vi "LV to ITX  Retrieve_SE mode  calculate R.vi"(0 "File or Folder Path":path=path "\\\\WINDYSEA\\Data/SA02835E.20160621/5_IV - sweep Bx, By, Vsg", 5 "offset":i32, 7 "length":i32=1, 9 "index":T2={"A"=3, "B"=7, "C"=5, "D"=7, "E"=3, "N1"=22, "N2"=2, "N3"=3, "N4"=4, "A 1"=8, "A 2"=10, "C 1"=5, "C 2"=1, "E 2"=4}, 11 "stop":bool=TRUE, 12 "file contains 2D data?":bool) -> (1 "Spherical coordinates":dbl[][](array[numeric]), 2 "long":cluster{i32[], dbl[]}(graph), 3 "G vs T":cluster{dbl[], dbl[]}(graph), 4 "A vs B":cluster{dbl[], dbl[]}[](graph), 6 "C vs D":cluster{dbl[], dbl[]}[](graph), 8 "E( = A)":dbl[][](graph), 10 "N":cluster{"N1":dbl, "N2":dbl, "N3":dbl, "N4":dbl}={"N1"=0.275, "N2"=1.998590895326537, "N3"=1.188236459055352e-05, "N4"=3.553800592300099e-05} {"N4" format="%#_6p"; "N3" format="%#_6p"; "N2" format="%#_6p"; "N1" format="%#_6p"}, 13 "Index, Wavenames":string[][](table)=[["0", "'time.SA02835E.20160621.000000'\n"], ["1", "'temp.SA02835E.20160621.000000'\n"], ["2", "'Bx.SA02835E.20160621.000000'\n"], ["3", "'By.SA02835E.20160621.000000'\n"], ["4", "'Bz.SA02835E.20160621.000000'\n"], ["5", "'Vsource.SA02835E.20160621.000000'\n"], ["6", "'Lockin0.SA02835E.20160621.000000'\n"], ["7", "'Lockin1.SA02835E.20160621.000000'\n"], ["8", "'Lockin2.SA02835E.20160621.000000'\n"], ["9", "'Lockin3.SA02835E.20160621.000000'\n"], ["10", "'Lockin4.SA02835E.20160621.000000'\n"], ["11", "'Lockin5.SA02835E.20160621.000000'\n"], ["12", "'Lockin6.SA02835E.20160621.000000'\n"], ["13", "'Lockin7.SA02835E.20160621.000000'\n"], ["14", "'B_rate.SA02835E.20160621.000000'\n"], ["15", "'DC0.SA02835E.20160621.000000'\n"], ["16", "'DC1.SA02835E.20160621.000000'\n"], ["17", "'DC2.SA02835E.20160621.000000'\n"], ["18", "'DC3.SA02835E.20160621.000000'\n"], ["19", "'DC4.SA02835E.20160621.000000'\n"], ["20", "'DC5.SA02835E.20160621.000000'\n"], ["21", "'DC6.SA02835E.20160621.000000'\n"], ["22", "'DC7.SA02835E.20160621.000000'\n"], ["23", "'V4T.SA02835E.20160621.000000'\n"], ["24", "'I.SA02835E.20160621.000000'\n"], ["", ""]], 14 "Comments":string="IGOR\nX// Date: 6/25/2016 8:10 PM\nX// sweep in plane: from theta=0 deg to 360 deg in 10 deg steps (phi=90, xy plane) @ 0.005 T/min\nX// sweep Vsg: -30mV to 275mV, 1mV steps\nX// \nX// taking lockin data between Bfield setpoints\nX// \nX// IV:\nX// low cutoff f: 0.01\nX// decimate: 10\nX// \nX// Vbg=0.57V\nX// \nX// lockin:\nX// 0: 27\nX// 1: 1 current, 3mV AC, 675uV DC, 0.4Hz\nX// 2: 2, \nX// 3: 6,\nX// 4: 7 \nX// 5: 8 current\nX// 6; 28 \nX// appliedVsg= -0.030000\n\n\n\n\n\n\n\n\n\n\n\n\n\n\n\n\n\n\n\n\n\n\n\n\n\n\n\n\n\n\n\n\n\n\n\n\n\n\n\n\n\n\n\n\n\n\n\n\n\n\n\n\nX \nX Display/R 'time.SA02835E.20160621.000000'\nX AppendToGraph 'temp.SA02835E.20160621.000000'\nX AppendToGraph 'Bx.SA02835E.20160621.000000'\nX AppendToGraph 'By.SA02835E.20160621.000000'\nX AppendToGraph 'Bz.SA02835E.20160621.000000'\nX AppendToGraph 'Vsource.SA02835E.20160621.000000'\nX AppendToGraph 'Lockin0.SA02835E.20160621.000000'\nX AppendToGraph 'Lockin1.SA02835E.20160621.000000'\nX AppendToGraph 'Lockin2.SA02835E.20160621.000000'\nX AppendToGraph 'Lockin3.SA02835E.20160621.000000'\nX AppendToGraph 'Lockin4.SA02835E.20160621.000000'\nX AppendToGraph 'Lockin5.SA02835E.20160621.000000'\nX AppendToGraph 'Lockin6.SA02835E.20160621.000000'\nX AppendToGraph 'Lockin7.SA02835E.20160621.000000'\nX AppendToGraph 'B_rate.SA02835E.20160621.000000'\nX AppendToGraph 'DC0.SA02835E.20160621.000000'\nX AppendToGraph 'DC1.SA02835E.20160621.000000'\nX AppendToGraph 'DC2.SA02835E.20160621.000000'\nX AppendToGraph 'DC3.SA02835E.20160621.000000'\nX AppendToGraph 'DC4.SA02835E.20160621.000000'\nX AppendToGraph 'DC5.SA02835E.20160621.000000'\nX AppendToGraph 'DC6.SA02835E.20160621.000000'\nX AppendToGraph 'DC7.SA02835E.20160621.000000'\nX AppendToGraph 'V4T.SA02835E.20160621.000000'\nX AppendToGraph 'I.SA02835E.20160621.000000'\nX Label bottom \"x label\"\nX Label left \"y label\"\nX ModifyGraph rgb('time.SA02835E.20160621.000000')=(65280,0,0)\nX ModifyGraph rgb('temp.SA02835E.20160621.000000')=(65280,13824,0)\nX ModifyGraph rgb('Bx.SA02835E.20160621.000000')=(65280,27648,0)\nX ModifyGraph rgb('By.SA02835E.20160621.000000')=(65280,43008,0)\nX ModifyGraph rgb('Bz.SA02835E.20160621.000000')=(65280,56832,0)\nX ModifyGraph rgb('Vsource.SA02835E.20160621.000000')=(60416,65280,0)\nX ModifyGraph rgb('Lockin0.SA02835E.20160621.000000')=(46592,65280,0)\nX ModifyGraph rgb('Lockin1.SA02835E.20160621.000000')=(32768,65280,0)\nX ModifyGraph rgb('Lockin2.SA02835E.20160621.000000')=(17408,65280,0)\nX ModifyGraph rgb('Lockin3.SA02835E.20160621.000000')=(3584,65280,0)\nX ModifyGraph rgb('Lockin4.SA02835E.20160621.000000')=(0,65280,10240)\nX ModifyGraph rgb('Lockin5.SA02835E.20160621.000000')=(0,65280,24064)\nX ModifyGraph rgb('Lockin6.SA02835E.20160621.000000')=(0,65280,37888)\nX ModifyGraph rgb('Lockin7.SA02835E.20160621.000000')=(0,65280,53248)\nX ModifyGraph rgb('B_rate.SA02835E.20160621.000000')=(0,64000,65280)\nX ModifyGraph rgb('DC0.SA02835E.20160621.000000')=(0,50176,65280)\nX ModifyGraph rgb('DC1.SA02835E.20160621.000000')=(0,36352,65280)\nX ModifyGraph rgb('DC2.SA02835E.20160621.000000')=(0,22528,65280)\nX ModifyGraph rgb('DC3.SA02835E.20160621.000000')=(0,7168,65280)\nX ModifyGraph rgb('DC4.SA02835E.20160621.000000')=(6656,0,65280)\nX ModifyGraph rgb('DC5.SA02835E.20160621.000000')=(20480,0,65280)\nX ModifyGraph rgb('DC6.SA02835E.20160621.000000')=(34304,0,65280)\nX ModifyGraph rgb('DC7.SA02835E.20160621.000000')=(48128,0,65280)\nX ModifyGraph rgb('V4T.SA02835E.20160621.000000')=(63488,0,65280)\nX ModifyGraph rgb('I.SA02835E.20160621.000000')=(65280,0,53760)\nX Legend/C/N=text0/J \"\\\\s('time.SA02835E.20160621.000000') time\\r\\\\s('temp.SA02835E.20160621.000000') temp\\r\\\\s('Bx.SA02835E.20160621.000000') Bx\\r\\\\s('By.SA02835E.20160621.000000') By\\r\\\\s('Bz.SA02835E.20160621.000000') Bz\\r\\\\s('Vsource.SA02835E.20160621.000000') Vsource\\r\\\\s('Lockin0.SA02835E.20160621.000000') Lockin0\\r\\\\s('Lockin1.SA02835E.20160621.000000') Lockin1\\r\\\\s('Lockin2.SA02835E.20160621.000000') Lockin2\\r\\\\s('Lockin3.SA02835E.20160621.000000') Lockin3\\r\\\\s('Lockin4.SA02835E.20160621.000000') Lockin4\\r\\\\s('Lockin5.SA02835E.20160621.000000') Lockin5\\r\\\\s('Lockin6.SA02835E.20160621.000000') Lockin6\\r\\\\s('Lockin7.SA02835E.20160621.000000') Lockin7\\r\\\\s('B_rate.SA02835E.20160621.000000') B_rate\\r\\\\s('DC0.SA02835E.20160621.000000') DC0\\r\\\\s('DC1.SA02835E.20160621.000000') DC1\\r\\\\s('DC2.SA02835E.20160621.000000') DC2\\r\\\\s('DC3.SA02835E.20160621.000000') DC3\\r\\\\s('DC4.SA02835E.20160621.000000') DC4\\r\\\\s('DC5.SA02835E.20160621.000000') DC5\\r\\\\s('DC6.SA02835E.20160621.000000') DC6\\r\\\\s('DC7.SA02835E.20160621.000000') DC7\\r\\\\s('V4T.SA02835E.20160621.000000') V4T\\r\\\\s('I.SA02835E.20160621.000000') I\"\nX ModifyGraph mirror(bottom)=1\nX ModifyGraph width=216\nX ModifyGraph height={Aspect,0.6}\nX ModifyGraph Log(bottom)=0\nX ModifyGraph Log(left)=0\nX \n", 15 "E index vs Field":cluster{i32[], dbl[]}(graph))   [LabVIEW 2016]
uses:
  <vilib>/Utility/miscctls.llb/LVOffsetAndMultiplierTypeDef.ctl
  <vilib>/Analysis/3filter.llb/Savitzky-Golay Filter (DBL).vi
  <vilib>/Analysis/2dsp.llb/Decimate (single shot, DBL).vi
  <vilib>/Analysis/NI_AALPro.lvlib
  <vilib>/Analysis/NI_AALBase.lvlib
panel:
  out "A or C vs N3":cluster{dbl[], dbl[]}[](graph)
  in  "A":bool
  in  "VRM mode":bool
  in  "Ring":u16(ring) items=["default", "DIFF"]
  in  "decimating factor":i32=1
  in  "decimate files":i32=1
  in  "side points":i32=6
  in  "fit points":dbl=10.0
  in  "dy/dx vs x":bool=TRUE
  in  "Portion of data":cluster{dbl, dbl}(slide)={0.75, 0.25} scale=0.0..1.0
  in  "length 2":i32=498
  in  "index 2":i32=72
  out "Ns":T1(array[cluster])
  in  "SE?":bool=TRUE
  in  "D  is time?":bool
  in  "B is time?":bool
  out "time":string[][](table)=[["6/25/2016", "8:10 PM"]]
  in  "Use Folder Index File?":bool
  in  "Generate Folder Index File?":bool
  in  "Ez name":string="Conductance (S)"
  in  "Ey name":string="BY (T)"
  in  "Ex name":string="Vsg (mV)"
  in  "C y name":string="voltage"
  in  "D x name":string="Vsg"
  in  "A y name":string="current"
  in  "B x name":string="Vsg"
  in  "recolor traces?":bool
  in  "Ex":T3={"Offset"=0.0, "Multiplier"=1.0}
  in  "Ey":T3={"Offset"=0.0, "Multiplier"=1.0}
  out "Path":path=path "\\\\WINDYSEA\\Data/SA02835E.20160621/5_IV - sweep Bx, By, Vsg/SA02835E.20160621.000000.itx"
  out "counter":i32
  in  "pattern":string="*.itx"
  # "A1-A2\nC1-C2\nE-E2"
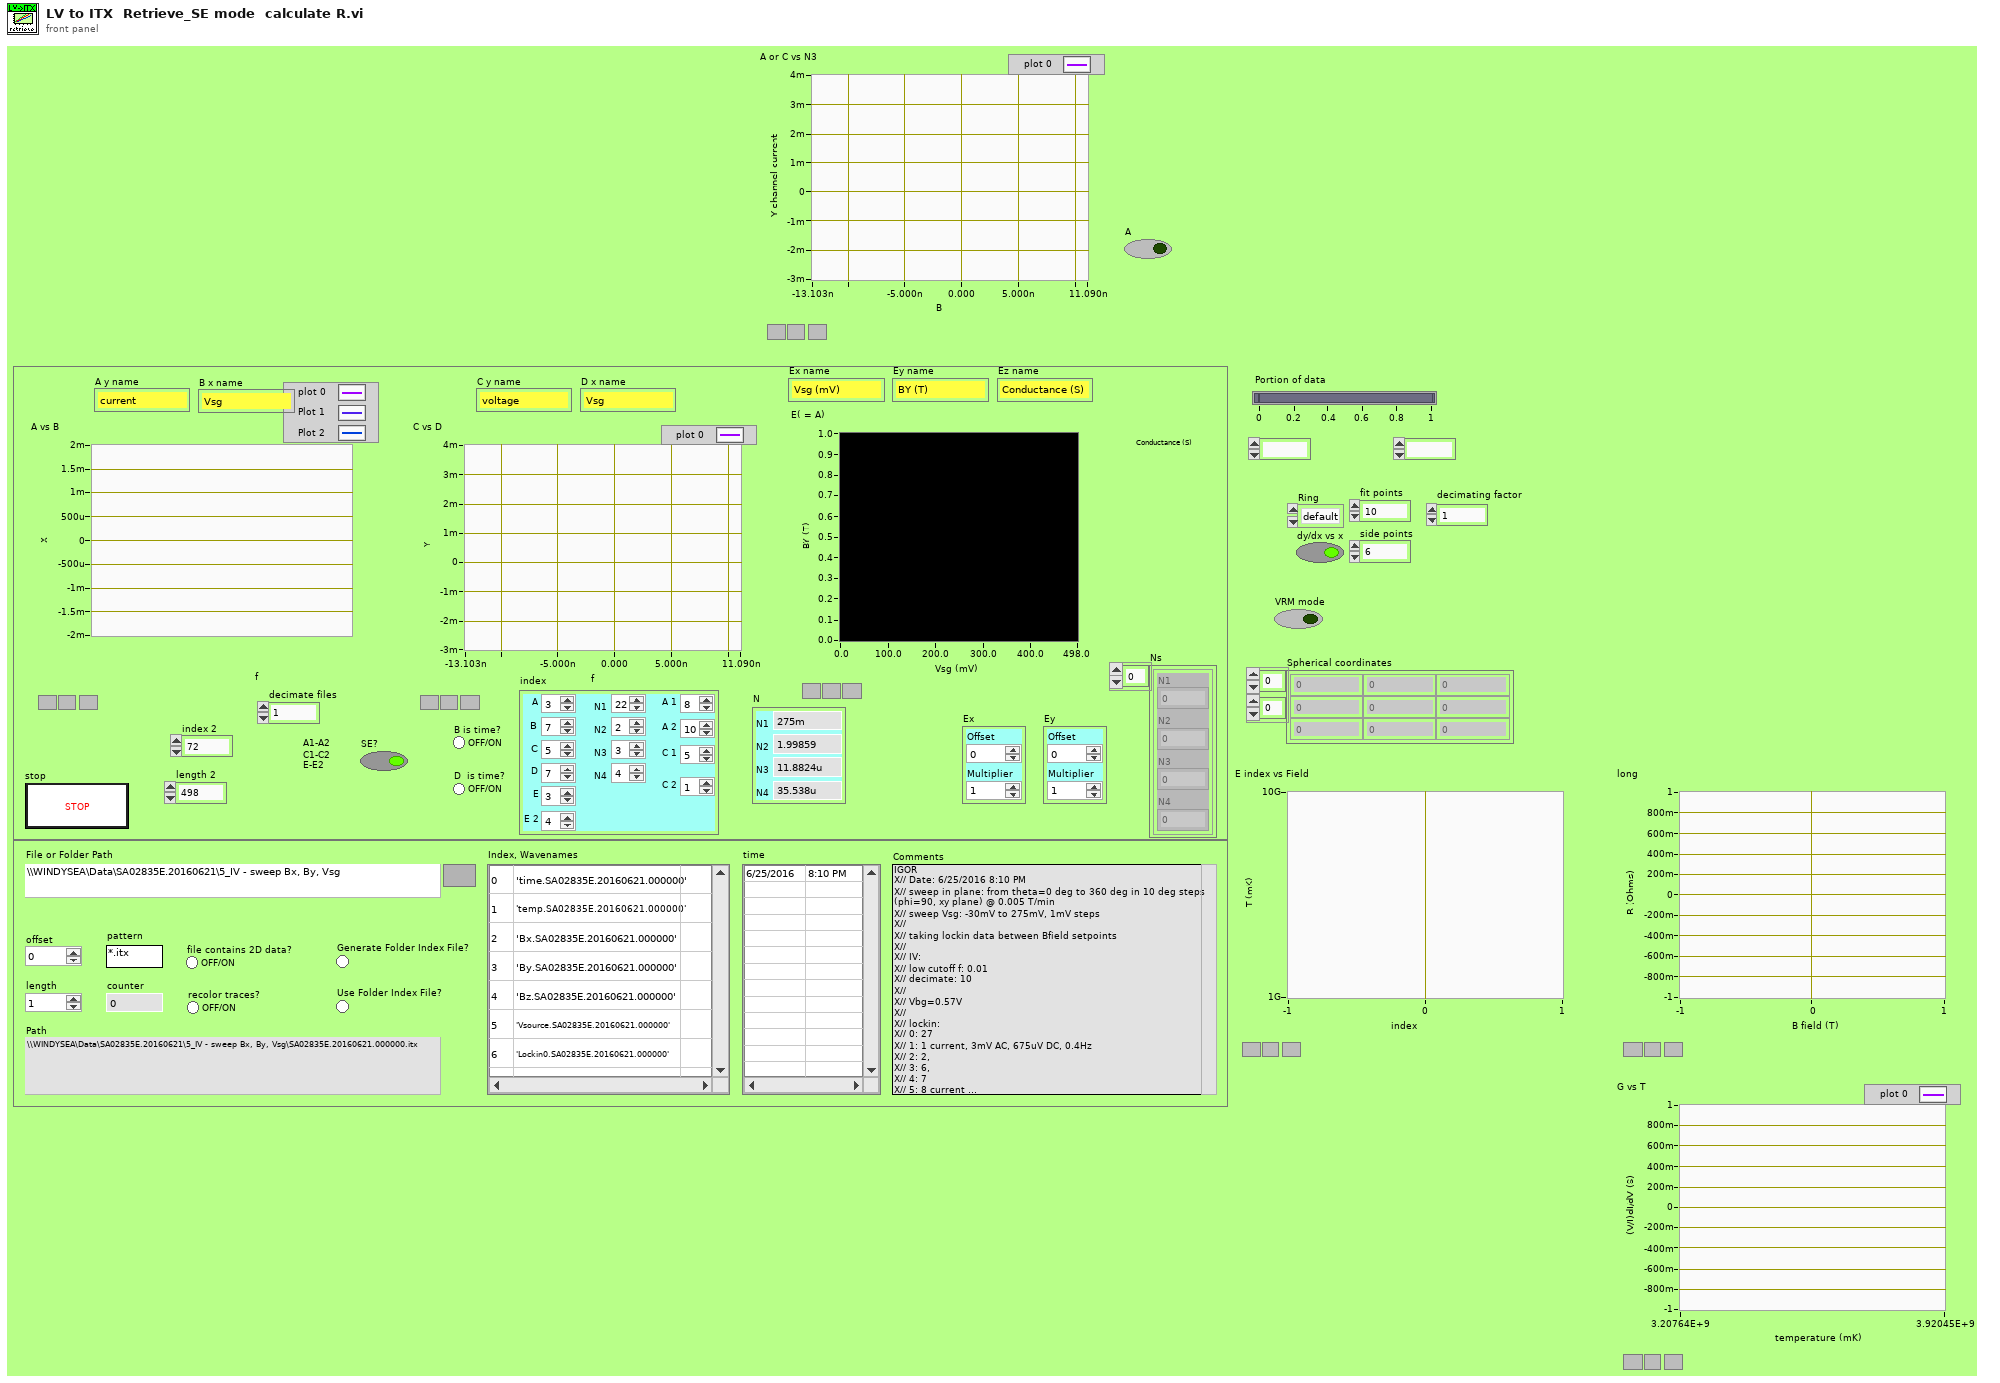
[diagram p1: front panel]
types:
  T1 = cluster{"N1":dbl, "N2":dbl, "N3":dbl, "N4":dbl}[]
  T2 = cluster{"A":i32, "B":i32, "C":i32, "D":i32, "E":i32, "N1":i32, "N2":i32, "N3":i32, "N4":i32, "A 1":i32, "A 2":i32, "C 1":i32, "C 2":i32, "E 2":i32}
  T3 = typedef "LVOffsetAndMultiplierTypeDef.ctl" = cluster{"Offset":dbl, "Multiplier":dbl}
  T4 = cluster{"Decimated Array":dbl[], "Decimated Array":dbl[]}
  T5 = cluster{"Decimated Array":dbl[], "Filtered X":dbl[]}
  T6 = cluster{"Decimated Array":dbl[], "Filtered X":dbl[]}[]
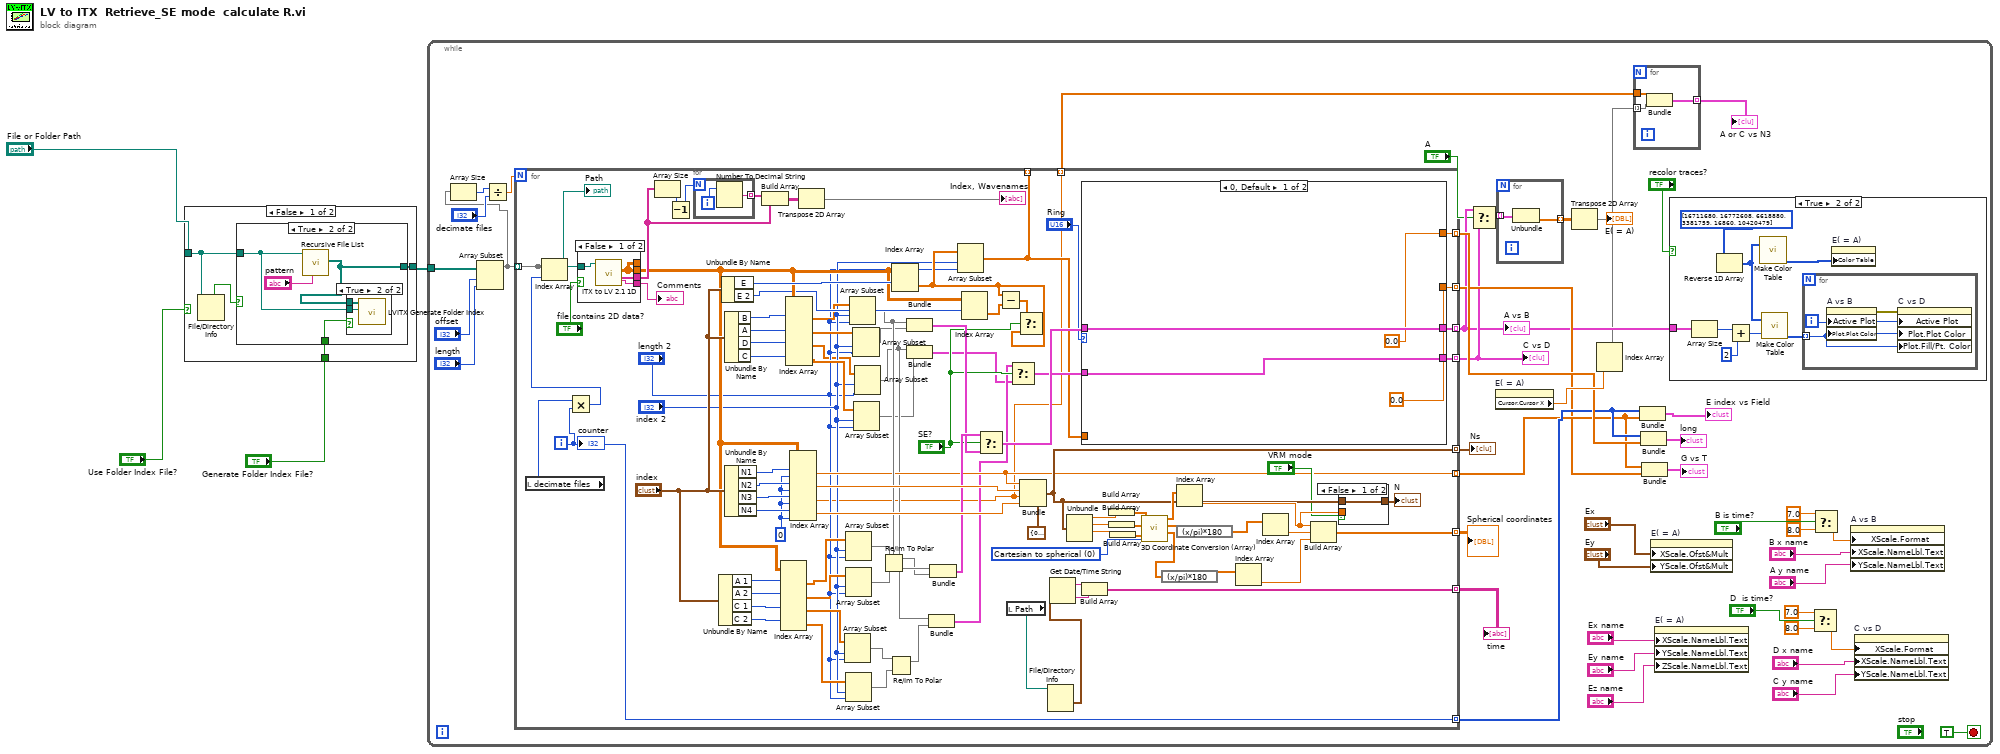
[diagram p0: block diagram]
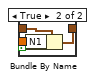
[diagram p3: hidden frame]
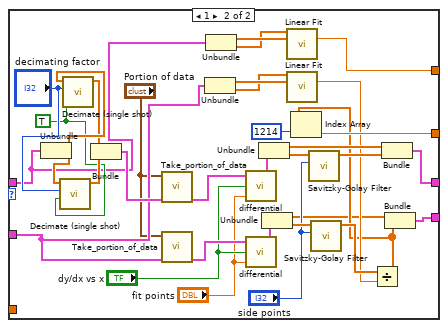
[diagram p4: hidden frame]
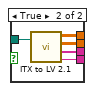
[diagram p5: hidden frame]
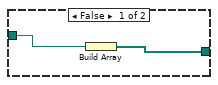
[diagram p6: hidden frame]
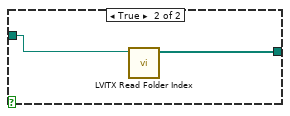
[diagram p8: hidden frame]
diagram:
  n1 = case shown="False" "Use Folder Index File?" {
    tunnel: [w6 w17] -> w2
    tunnel: "File or Folder Path" -> [w8 w18]
    tunnel: "Generate Folder Index File?" -> [w5 _]
    frame False {
      n2 = File/Directory Info(path=w8) -> (directory=w7:bool)  [unwired: 1 in, 6 out]
      n3 = case shown="True" w7 {
        tunnel: [w10 w13] -> w6
        tunnel: w8 -> [w9 w12]
        tunnel: w5 -> [_ w11]
        frame False {
          n4 = Build Array(w9) -> (w10:path[])
        }
        frame True {
          n5 = call <vilib>:"Recursive File List.vi"("pattern"="pattern", "Folder Path"=w12) -> ("All Files in Dir"=w13:path[])  [unwired: 5 in, 4 out]
          n6 = case shown="True" w11 {
            tunnel: w13 -> [_ w16]
            tunnel: w12 -> [_ w15]
            frame False {
            }
            frame True {
              n7 = call <userlib>:"LVITX Generate Folder Index.vi"("File or Folder Path"=w15, "All Files in Dir"=w16) -> ()  [unwired: 10 in]
            }
          }
        }
      }
    }
    frame True {
      n8 = call <userlib>:"LVITX Read Folder Index.vi"("File or Folder Path"=w18) -> ("Array"=w17:path[])  [unwired: 10 in]
    }
  }
  n9 = while {
    tunnel: w2 -> [w40]
    stop <- TRUE stop-if-true
    n10 = Array Subset(array=w40, index="offset", length="length") -> (w36:path[])
    n11 = Array Size(array=w36) -> (size(s)=w39:i32)
    n12 = Divide(x=w39, y="decimate files") -> (x/y=w37:dbl)
    n13 = for {
      N: w37 -> [_]
      tunnel: w36 -> [w173]
      tunnel: [w173] -> _ mode=indexing
      tunnel: [w111] -> w23 mode=indexing
      tunnel: [w110] -> w24 mode=indexing
      tunnel: [w149] -> w54 mode=indexing
      tunnel: [w100] -> w43 mode=indexing
      tunnel: [w109] -> w41 mode=indexing
      tunnel: [w103] -> w33 mode=indexing
      tunnel: [w102] -> w26 mode=indexing
      tunnel: [w97] -> w29 mode=indexing
      tunnel: [w96] -> w28 mode=indexing
      tunnel: [w81] -> _ mode=indexing
      tunnel: [w80] -> w20 mode=indexing
      i -> [w97]
      w126 = u16 0 items=["Cartesian to spherical", "spherical to Cartesian", "Cartesian to cylindrical", "cylindrical to Cartesian", "spherical to cylindrical", "cylindrical to spherical"] ("conversion type")
      w147 = 0 ("disabled index (col)")
      n14 = local read "decimate files"() -> (w106:i32)
      n15 = Multiply(x=w106, y=w97) -> (x*y=w107:i32)
      n16 = Index Array(array=w173, index=w107) -> (element=w108:path)
      "Path" <- w108
      n17 = case shown="False" "file contains 2D data?" {
        tunnel: [w222 w225] -> w174
        tunnel: [w220 w226] -> w139
        tunnel: w108 -> [w221 w227]
        tunnel: [w219 w224] -> w166
        tunnel: [w220 w223] -> _
        frame False {
          n18 = call <userlib>:"ITX to LV 2.1 1D.vi"("file (use dialog)"=w221) -> ("wave names"=w219:string[], "1D arrays"=w220:dbl[][], "Notes"=w222:string)  [unwired: 6 in, 2 out]
        }
        frame True {
          n19 = call <userlib>:"ITX to LV 2.1.vi"("file (use dialog)"=w227) -> ("2D array"=w223:dbl[][], "1D arrays"=w226:dbl[][], "wave names"=w224:string[], "Notes"=w225:string)  [unwired: 1 in]
        }
      }
      "Comments" <- w174
      n20 = Array Size(array=w166) -> (size(s)=w169:i32)
      n21 = Decrement(x=w169) -> (x-1=w168:i32)
      n22 = for {
        N: w168 -> [_]
        tunnel: [w217] -> w171 mode=indexing
        i -> [w218]
        n23 = Number To Decimal String(number=w218) -> (decimal integer string=w217:string)  [unwired: 1 in]
      }
      n24 = Unbundle By Name("index") -> ("A 1"=w146:i32, "A 2"=w145:i32, "C 1"=w144:i32, "C 2"=w143:i32)
      n25 = Unbundle By Name("index") -> ("E"=w159:i32, "E 2"=w138:i32)
      n26 = Unbundle By Name("index") -> ("B"=w158:i32, "A"=w157:i32, "D"=w156:i32, "C"=w155:i32)
      n27 = Unbundle By Name("index") -> ("N1"=w160:i32, "N2"=w161:i32, "N3"=w162:i32, "N4"=w163:i32)
      n28 = Build Array(w171, w166) -> (w167:string[][])
      n29 = Index Array(array=w139, index (row) #1=w146, index (row) #2=w145, index (row) #3=w144, index (row) #4=w143) -> (element #1=w130:dbl[], element #2=w129:dbl[], element #3=w128:dbl[], element #4=w127:dbl[])  [unwired: 4 in]
      n30 = Index Array(array=w139, index (row) #1=w158, index (row) #2=w157, index (row) #3=w156, index (row) #4=w155) -> (element #1=w135:dbl[], element #2=w133:dbl[], element #3=w89:dbl[], element #4=w131:dbl[])  [unwired: 4 in]
      n31 = Index Array(array=w139, index (row) #1=w160, index (col) #1=w147, index (row) #2=w161, index (col) #2=w147, index (row) #3=w162, index (col) #3=w147, index (row) #4=w163, index (col) #4=w147) -> (element #1=w96:dbl, element #2=w153:dbl, element #3=w80:dbl, element #4=w165:dbl)
      n32 = Transpose 2D Array(2D array=w167) -> (transposed array=→"Index, Wavenames":string[][])
      n33 = Array Subset(array=w128, index="index 2", length="length 2") -> (w84:dbl[])
      n34 = Array Subset(array=w130, index="index 2", length="length 2") -> (w87:dbl[])
      n35 = Array Subset(array=w129, index="index 2", length="length 2") -> (w86:dbl[])
      n36 = Array Subset(array=w127, index="index 2", length="length 2") -> (w83:dbl[])
      n37 = Array Subset(array=w135, index="index 2", length="length 2") -> (w134:dbl[])
      n38 = Array Subset(array=w133, index="index 2", length="length 2") -> (w132:dbl[])
      n39 = Array Subset(array=w131, index="index 2", length="length 2") -> (w88:dbl[])
      n40 = Array Subset(array=w89, index="index 2", length="length 2") -> (w90:dbl[])
      n41 = Re/Im To Polar(2:w86, 3:w87) -> (1:w85:dbl[])  [unwired: 1 out]
      n42 = Re/Im To Polar(2:w83, 3:w84) -> (1:w82:dbl[])  [unwired: 1 out]
      n43 = Index Array(array=w139, index (row)=w159) -> (element=w93:dbl[])  [unwired: 1 in]
      n44 = Bundle(w134, w132) -> (w141:cluster{dbl[], dbl[]})  [unwired: 1 in]
      n45 = Bundle(w90, w88) -> (w94:cluster{dbl[], dbl[]})  [unwired: 1 in]
      n46 = Bundle(w90, w82) -> (w95:cluster{dbl[], dbl[]})  [unwired: 1 in]
      n47 = Bundle(w134, w85) -> (w142:cluster{dbl[], dbl[]})  [unwired: 1 in]
      n48 = Array Subset(array=w93, index="index 2", length="length 2") -> (w81:dbl[])
      n49 = Index Array(array=w139, index (row)=w138) -> (element=w137:dbl[])  [unwired: 1 in]
      n50 = Select(t=w142, s="SE?", f=w141) -> (s? t:f=w113:cluster{dbl[], dbl[]})
      n51 = Subtract(x=w93, y=w137) -> (x-y=w136:dbl[])
      n52 = local read "Path"() -> (w154:path)
      n53 = Select(t=w95, s="SE?", f=w94) -> (s? t:f=w112:cluster{dbl[], dbl[]})
      n54 = Select(t=w136, s="SE?", f=w93) -> ()  [unwired: 1 out]
      n55 = Bundle(cluster=cluster{"N1":dbl, "N2":dbl, "N3":dbl, "N4":dbl} {"N1"=0.0, "N2"=0.0, "N3"=0.0, "N4"=0.0}, "N1"=w96, "N2"=w153, "N3"=w80, "N4"=w165) -> (w100:cluster{"N1":dbl, "N2":dbl, "N3":dbl, "N4":dbl})
      n56 = File/Directory Info(path=w154) -> (last mod=w152:timestamp)  [unwired: 1 in, 6 out]
      n57 = Get Date/Time String(seconds (now)=w152) -> (date string=w151:string, time string=w150:string)  [unwired: 2 in]
      n58 = Unbundle(w100) -> ("N1"=w105:dbl, "N2"=w125:dbl, "N3"=w122:dbl)  [unwired: 1 out]
      n59 = case shown="0, Default" "Ring" {
        tunnel: w113 -> [w182 w200]
        tunnel: w112 -> [w181 w189]
        tunnel: [w182 w185] -> w111
        tunnel: [w181 w184] -> w110
        tunnel: [0.0 w197] -> w103
        tunnel: [0.0 w194] -> w102
        tunnel: w81 -> [_ _]
        frame 0, Default {
        }
        frame 1 {
          w201 = TRUE ("averaging")
          n60 = Unbundle(w200) -> (w206:dbl[], w204:dbl[])
          n61 = call-poly <vilib>:"Decimate (single shot).vi"("averaging"=w201, "decimating factor"="decimating factor", "X"=w204) -> ("Decimated Array"=w203:dbl[])  [unwired: 7 in, 1 out]
          n62 = call-poly <vilib>:"Decimate (single shot).vi"("averaging"=w201, "decimating factor"="decimating factor", "X"=w206) -> ("Decimated Array"=w205:dbl[])  [unwired: 7 in, 1 out]
          n63 = Bundle("Decimated Array"=w205, "Decimated Array"=w203) -> (w207:T4)  [unwired: 1 in]
          n64 = call <userlib>:"Take_portion_of_data.vi"("input IV"=w207, "Slide"="Portion of data") -> ("Output IV"=w215:cluster{dbl[], dbl[]})  [unwired: 5 in]
          n65 = call <userlib>:"Take_portion_of_data.vi"("input IV"=w189, "Slide"="Portion of data") -> ("Output IV"=w216:cluster{dbl[], dbl[]})  [unwired: 5 in]
          n66 = Unbundle(w189) -> (w198:dbl[], w193:dbl[])
          n67 = Unbundle(w200) -> (w199:dbl[], w196:dbl[])
          n68 = call <userlib>:"differential.vi"("Numeric"="fit points", "dy/dx vs x"="dy/dx vs x", "A vs B 2"=w215) -> ("A vs B 3"=w211:T4)  [unwired: 1 in]
          n69 = call <userlib>:"differential.vi"("Numeric"="fit points", "dy/dx vs x"="dy/dx vs x", "A vs B 2"=w216) -> ("A vs B 3"=w209:T4)  [unwired: 1 in]
          n70 = Unbundle(w211) -> ("Decimated Array"=w214:dbl[], "Decimated Array"=w212:dbl[])
          n71 = Unbundle(w209) -> ("Decimated Array"=w183:dbl[], "Decimated Array"=w210:dbl[])
          n72 = call <vilib>:"Linear Fit.vi"("Y"=w196, "X"=w199) -> ("slope"=w197:dbl)  [unwired: 9 in, 4 out]
          n73 = call <vilib>:"Linear Fit.vi"("Y"=w193, "X"=w198) -> ("slope"=w191:dbl)  [unwired: 9 in, 4 out]
          n74 = call-poly <vilib>:"Savitzky-Golay Filter.vi"("side points"="side points", "X"=w212) -> ("Filtered X"=w213:dbl[])  [unwired: 8 in, 1 out]
          n75 = call-poly <vilib>:"Savitzky-Golay Filter.vi"("side points"="side points", "X"=w210) -> ("Filtered X"=w192:dbl[])  [unwired: 8 in, 1 out]
          n76 = Divide(x=w192, y=w191) -> (x/y=w190:dbl[])
          n77 = Index Array(array=w190, index=1214) -> (element=w194:dbl)
          n78 = Bundle("Decimated Array"=w214, "Filtered X"=w213) -> (w185:T5)  [unwired: 1 in]
          n79 = Bundle("Decimated Array"=w183, w190) -> (w184:cluster{"Decimated Array":dbl[], dbl[]})  [unwired: 1 in]
        }
      }
      n80 = Build Array(w151, w150) -> (w149:string[])
      n81 = Build Array(w105) -> (w124:dbl[])
      n82 = Build Array(w125) -> (w123:dbl[])
      n83 = Build Array(w122) -> (w121:dbl[])
      n84 = call <vilib>:"3D Coordinate Conversion (Array).vi"("conversion type"=w126, "Axis 3"=w121, "Axis 2"=w123, "Axis 1"=w124) -> ("Axis 3 Out"=w119:dbl[], "Axis 2 Out"=w120:dbl[], "Axis 1 Out"=w118:dbl[])  [unwired: 4 in, 1 out]
      n85 = expression code="(x/pi)*180" ("degrees to radians")(w119) -> (w116:dbl[])
      n86 = Index Array(array=w118) -> (element=w101:dbl)  [unwired: 1 in]
      n87 = expression code="(x/pi)*180" ("degrees to radians")(w120) -> (w117:dbl[])
      n88 = Index Array(array=w116) -> (element=w114:dbl)  [unwired: 1 in]
      n89 = Index Array(array=w117) -> (element=w115:dbl)  [unwired: 1 in]
      n90 = Build Array(w101, w115, w114) -> (w109:dbl[])
      n91 = case shown="False" "VRM mode" {
        tunnel: w101 -> [_ w178]
        tunnel: w100 -> [w175 w177]
        tunnel: [w175 w176] -> w99
        frame False {
        }
        frame True {
          n92 = Bundle By Name(cluster=w177, "N1"=w178) -> (w176:cluster{"N1":dbl, "N2":dbl, "N3":dbl, "N4":dbl})
        }
      }
      "N" <- w99
      "counter" <- w97
    }
    "time" <- w54
    "Ns" <- w43
    "Spherical coordinates" <- w41
    "A vs B" <- w23
    "C vs D" <- w24
    n93 = Select(t=w23, s="A", f=w24) -> (s? t:f=w25:T6)
    n94 = property on="E( = A)" class="IntGraph (strict)"() -> ("Cursor.Cursor X"=w34:dbl)  [unwired: 2 in, 2 out]
    n95 = for {
      tunnel: [w68] -> w42 mode=indexing
      tunnel: [w67] -> _ mode=indexing
      tunnel: w25 -> [w67] mode=indexing
      n96 = Unbundle(w67) -> ("Filtered X"=w68:dbl[])  [unwired: 1 out]
    }
    n97 = Transpose 2D Array(2D array=w42) -> (transposed array=w21:dbl[][])
    "E( = A)" <- w21
    n98 = Index Array(array=w21, index (row)=w34) -> ()  [unwired: 1 in, 1 out]
    n99 = for {
      tunnel: w21 -> [w66] mode=indexing
      tunnel: w20 -> [w65]
      tunnel: [w64] -> w19 mode=indexing
      n100 = Bundle(w65, w66) -> (w64:cluster{dbl[], dbl[]})  [unwired: 1 in]
    }
    "A or C vs N3" <- w19
    n101 = Bundle(w29, w28) -> (→"E index vs Field":cluster{i32[], dbl[]})  [unwired: 1 in]
    n102 = Bundle(w29, w33) -> (→"long":cluster{i32[], dbl[]})  [unwired: 1 in]
    n103 = Bundle(w28, w26) -> (→"G vs T":cluster{dbl[], dbl[]})  [unwired: 1 in]
    n104 = property on="E( = A)" class="IntGraph (strict)"("XScale.Ofst&Mult"="Ex", "YScale.Ofst&Mult"="Ey") -> ()  [unwired: 2 in, 2 out]
    n105 = property on="E( = A)" class="IntGraph (strict)"("XScale.NameLbl.Text"="Ex name", "YScale.NameLbl.Text"="Ey name", "ZScale.NameLbl.Text"="Ez name") -> ()  [unwired: 2 in, 2 out]
    n106 = case shown="True" "recolor traces?" {
      tunnel: w23 -> [_ w71]
      frame False {
      }
      frame True {
        n107 = Array Size(array=w71) -> (size(s)=w72:i32)
        n108 = Reverse 1D Array(array=u32[] [16711680, 16772608, 6618880, 3381759, 16860, 10420479] ("color scale")) -> (reversed array=w70:u32[])
        n109 = Add(x=w72, y=2 ("x")) -> (x+y=w76:i32)
        n110 = call <userlib>:"Make Color Table.vi"("Array"=w70) -> ("Color Tbl"=w74:u32[])  [unwired: 1 in, 3 out]
        n111 = call <userlib>:"Make Color Table.vi"("Array"=w70, "Size/3"=w76) -> ("Color Tbl"=w73:u32[])  [unwired: 3 out]
        n112 = for {
          tunnel: w73 -> [w77] mode=indexing
          i -> [w78]
          n113 = property on="A vs B" class="XYGraph (strict)"("Active Plot"=w78, "Plot.Plot Color"=w77) -> (error out=w79:errorcluster)  [unwired: 2 in, 1 out]
          n114 = property on="C vs D" class="XYGraph (strict)"(error in=w79, "Active Plot"=w78, "Plot.Plot Color"=w77, "Plot.Fill/Pt. Color"=w77) -> ()  [unwired: 1 in, 2 out]
        }
        n115 = property on="E( = A)" class="IntGraph (strict)"("Color Table"=w74) -> ()  [unwired: 2 in, 2 out]
      }
    }
    n116 = Select(t=7.0, s="D  is time?", f=8.0) -> (s? t:f=w48:dbl)
    n117 = Select(t=7.0, s="B is time?", f=8.0) -> (s? t:f=w49:dbl)
    n118 = property on="A vs B" class="XYGraph (strict)"("XScale.Format"=w49, "XScale.NameLbl.Text"="B x name", "YScale.NameLbl.Text"="A y name") -> ()  [unwired: 2 in, 2 out]
    n119 = property on="C vs D" class="XYGraph (strict)"("XScale.Format"=w48, "XScale.NameLbl.Text"="D x name", "YScale.NameLbl.Text"="C y name") -> ()  [unwired: 2 in, 2 out]
  }
